vi "PropertyListAddVirtual.vi"(10 "vi reference":refnum<vi>, 11 "Property List in":refnum<vi>) -> (3 "Property List out":refnum<vi>)   [LabVIEW 2019, in "VIPropertyPicker.lvlib"]
uses:
  VIPropertyPicker.lvlib
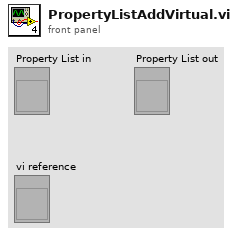
[diagram p1: front panel]
types:
  T1 = enum32{"Invalid", "Standard", "Closed", "Hidden", "Minimized", "Maximized"}
  T2 = typedef "LVRectTypeDef.ctl" = cluster{"Left":i16, "Top":i16, "Right":i16, "Bottom":i16}
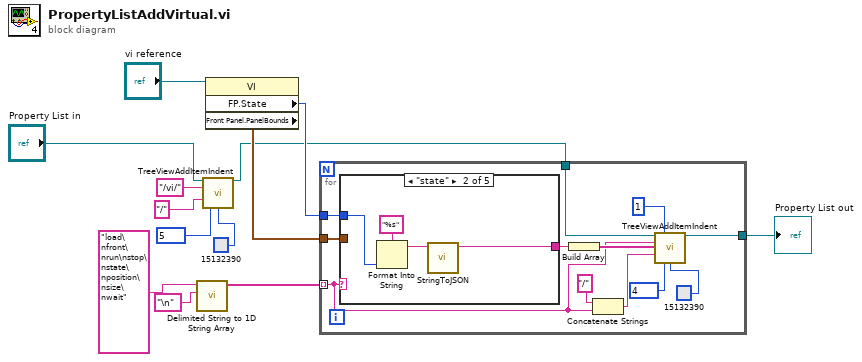
[diagram p0: block diagram]
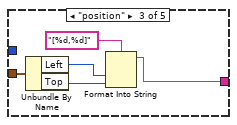
[diagram p3: hidden frame]
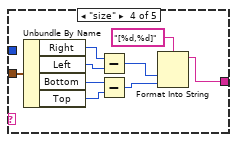
[diagram p4: hidden frame]
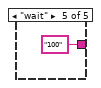
[diagram p5: hidden frame]
diagram:
  n1 = call <vilib>:"Delimited String to 1D String Array.vi"("delimiter"="\n", "delimited string"="load\nfront\nrun\nstop\nstate\nposition\nsize\nwait") -> ("string array"=w10:string[])  [unwired: 9 in]
  n2 = call "TreeViewAddItemIndent.vi"("TreeControl in"="Property List in", "Left Cell String"="/vi/", "Tag"="/", "Symbol Index"=5, "Background Color"=u32 15132390) -> ("TreeControl out"=w3:refnum<vi>)  [unwired: 8 in, 2 out]
  n3 = property class="VI"(reference="vi reference") -> ("FP.State"=w12:T1, "Front Panel.PanelBounds"=w13:T2)  [unwired: 1 in, 2 out]
  n4 = for {
    tunnel: w10 -> [w18] mode=indexing
    tunnel: w12 -> [w24]
    tunnel: w13 -> [w23]
    tunnel: w3 -> [w17]
    tunnel: [w16] -> w2
    n5 = case shown="\"state\"" w18 {
      tunnel: w24 -> [_ w29 _ _ _]
      tunnel: w23 -> [_ _ w34 w43 _]
      tunnel: [_ w26 w30 w41 "100" ("JSON string")] -> w22
      frame Default {
      }
      frame "state" {
        n6 = Format Into String(format string="%s", w29) -> (resulting string=w27:string)  [unwired: 2 in, 1 out]
        n7 = call "StringToJSON.vi"("input text"=w27) -> ("JSON string"=w26:string)  [unwired: 10 in]
      }
      frame "position" {
        n8 = Unbundle By Name(w34) -> ("Left"=w33:i16, "Top"=w32:i16)
        n9 = Format Into String(format string="[%d,%d]", w33, w32) -> (resulting string=w30:string)  [unwired: 2 in, 1 out]
      }
      frame "size" {
        n10 = Unbundle By Name(w43) -> ("Right"=w39:i16, "Left"=w40:i16, "Bottom"=w37:i16, "Top"=w36:i16)
        n11 = Subtract(x=w39, y=w40) -> (x-y=w38:i16)
        n12 = Subtract(x=w37, y=w36) -> (x-y=w35:i16)
        n13 = Format Into String(format string="[%d,%d]", w38, w35) -> (resulting string=w41:string)  [unwired: 2 in, 1 out]
      }
      frame "wait" {
      }
    }
    n14 = Build Array(w22) -> (w21:string[])
    n15 = Concatenate Strings("/" ("string"), w18) -> (w19:string)
    n16 = call "TreeViewAddItemIndent.vi"("TreeControl in"=w17, "Indentation"=1, "Left Cell String"=w18, "Child Text"=w21, "Tag"=w19, "Symbol Index"=4, "Background Color"=u32 15132390) -> ("TreeControl out"=w16:refnum<vi>)  [unwired: 6 in, 2 out]
  }
  "Property List out" <- w2
